vi "Read Table_Ref.vi"(8 "error in (no error)":errorcluster, 11 "Multimeter in":refnum<class "Multimeter.lvclass">) -> (0 "error out":errorcluster, 2 "Table_Ref":refnum<vi>, 3 "Multimeter out":refnum<class "Multimeter.lvclass">)   [LabVIEW 2019, in "Multimeter.lvlib" / "Multimeter.lvclass"]
uses:
  Library/Multimeter.lvclass
  Library/Multimeter.lvclass/Multimeter.ctl
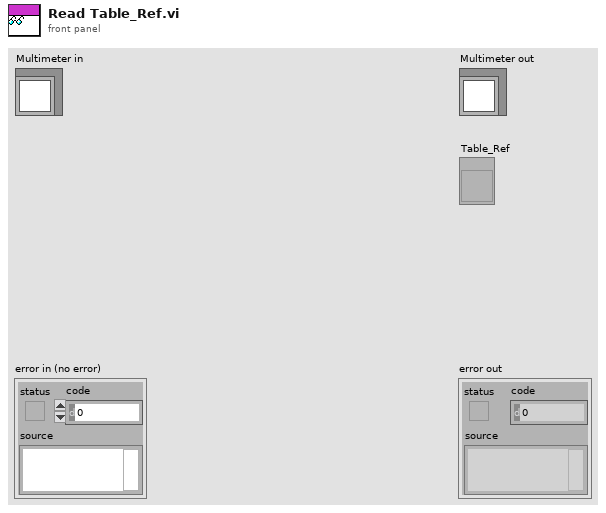
[diagram p1: front panel]
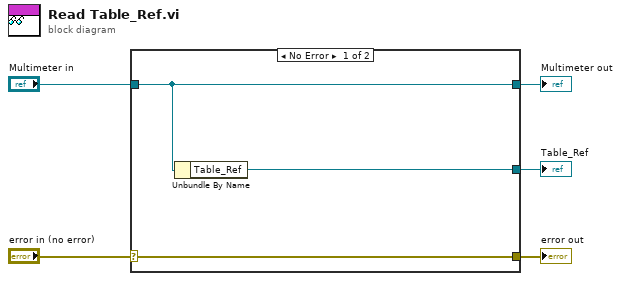
[diagram p0: block diagram]
diagram:
  n1 = case shown="No Error" "error in (no error)" {
    selector: "error in (no error)" -> [w8 w9]
    tunnel: [w8 w9] -> w4
    tunnel: [w7 w10] -> w2
    tunnel: "Multimeter in" -> [w7 w10]
    tunnel: [w6 _] -> w1
    frame No Error {
      n2 = Unbundle By Name(w7) -> ("Table_Ref"=w6:refnum<vi>)
    }
    frame Error {
    }
  }
  "error out" <- w4
  "Multimeter out" <- w2
  "Table_Ref" <- w1
